vi "二值化.vi"() -> (1 "确定":bool, 2 "数值":u8, 3 "方法":i32(ring) items=["clustering", "entropy", "metric", "moments", "inter-class variance"], 5 "自动":bool)   [LabVIEW 2018]
panel:
  in  "方法":i32(ring) items=["clustering", "entropy", "metric", "moments", "inter-class variance"]
  in  "自动":bool
  in  "确定":bool
  in  "滑动杆":u8(slide) scale=0.0..255.0
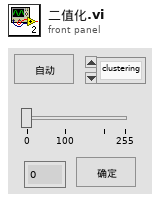
[diagram p1: front panel]
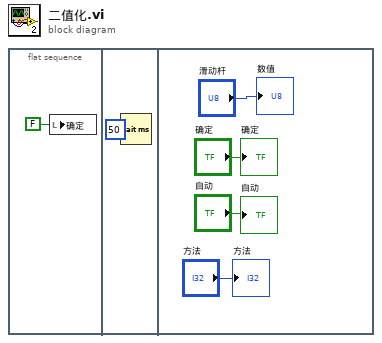
[diagram p0: block diagram]
diagram:
  n1 = flat-sequence {
    frame #0 {
      n2 = local write "确定"(FALSE ("确定")) -> ()
    }
    frame #1 {
      n3 = Wait (ms)(milliseconds to wait=u32 50 ("等待时间（毫秒）")) -> ()  [unwired: 1 out]
    }
    frame #2 {
      "数值" <- "滑动杆"
      "确定" <- "确定"
      "自动" <- "自动"
      "方法" <- "方法"
    }
  }
